vi "StateSelectionString.vi"(1 "Disallowed States":bool[](array[boolean]), 2 "State Triggers":bool[](array[boolean]), 3 "State Names":string[](array[string])) -> (0 "Selected State":string)   [LabVIEW 2019]
doc: "This VI is designed to convert (possibly conflicting) button presses (or other triggers) into a robot state string. While the triggers do not have to be instantaneous, you should design your human interfaces to never latch any state selection buttons. Disallowing states is also supported. If a state is allowed after not previously being allowed, the state trigger must be reissued."
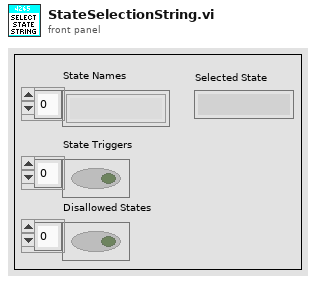
[diagram p1: front panel]
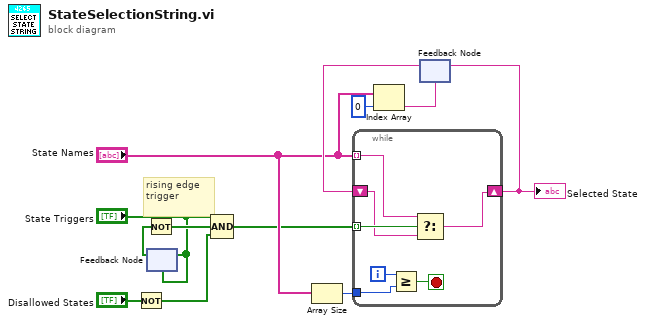
[diagram p0: block diagram]
diagram:
  # "rising edge\ntrigger"
  n1 = Not(x="Disallowed States") -> (.not. x?=w2:bool[])
  n2 = feedback #1("State Triggers") -> (w11:bool[])
  n3 = Not(x=w11) -> (.not. x?=w12:bool[])
  n4 = feedback-in #1("State Triggers") -> ()
  n5 = Compound Arithmetic op=AND("State Triggers", w12, w2) -> (w1:bool[])
  n6 = Array Size(array="State Names") -> (size(s)=w5:i32)
  n7 = Index Array(array="State Names", index=0) -> (element=w9:string)
  n8 = feedback #2(w9) -> (w8:string)
  n9 = while {
    tunnel: w1 -> [w19] mode=indexing
    tunnel: "State Names" -> [w17] mode=indexing
    shift-right: [w16] -> w7
    shift-left: w8 -> [w18]
    tunnel: w5 -> [w14]
    i -> [w15]
    stop <- w13 stop-if-true
    n10 = Greater Or Equal?(x=w15, y=w14) -> (x >= y?=w13:bool)
    n11 = Select(t=w17, s=w19, f=w18) -> (s? t:f=w16:string)
  }
  "Selected State" <- w7
  n12 = feedback-in #2(w7) -> ()
